vi "Date Lookup.vi"(10 "End Time Stamp":timestamp, 11 "Start Time Stamp":timestamp) -> (2 "Number of Days":i32, 3 "DateTime Array":timestamp[](array[timestamp]))   [LabVIEW 2012]
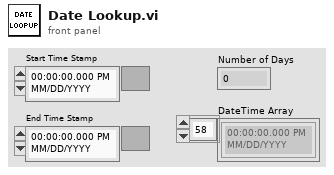
[diagram p1: front panel]
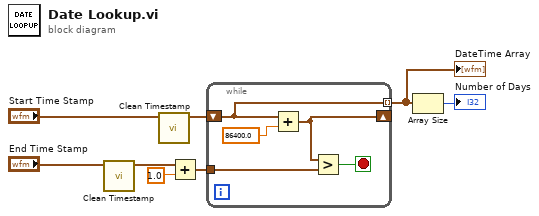
[diagram p0: block diagram]
diagram:
  n1 = call "Clean Timestamp.vi"("Time Stamp"="End Time Stamp") -> ("Clean time stamp"=w5:timestamp)  [unwired: 10 in]
  n2 = call "Clean Timestamp.vi"("Time Stamp"="Start Time Stamp") -> ("Clean time stamp"=w6:timestamp)  [unwired: 10 in]
  n3 = Add(x=w5, y=1.0) -> (x+y=w4:timestamp)
  n4 = while {
    tunnel: w4 -> [w12]
    shift-right: [w10] -> _
    shift-left: w6 -> [w9]
    tunnel: [w9] -> w2 mode=indexing
    stop <- w11 stop-if-true
    n5 = Add(x=w9, y=86400.0) -> (x+y=w10:timestamp)
    n6 = Greater?(x=w10, y=w12) -> (0:w11:bool)
  }
  "DateTime Array" <- w2
  n7 = Array Size(array=w2) -> (size(s)=→"Number of Days":i32)
